vi "receiver.vi"() -> ()   [LabVIEW 2013]
uses:
  <instrlib>/niUSRP/niUSRP Fetch Rx Data (CDB WDT).vi
  <vilib>/express/express analysis/Spectral/Block/exnSpectralBlock spectral measurements RMS poly.vi
  <vilib>/express/express analysis/Spectral/Block/exnSpectralBlock spectral measurements RMS WFM.vi
  <vilib>/express/express analysis/Spectral/XNode/ExpressSpectralMeasurementsBlockNode.xnode
panel:
  out "Waveform Graph 2":cluster{"f0":dbl, "df":dbl, "magnitude":dbl[]}(graph)
  out "Waveform Graph":waveform(dbl)[](graph)
  in  "stop":bool
  out "error out":errorcluster
  in  "number of samples":i64=1000
  out "coerced gain":dbl format="%#_6f"
  out "coerced carrier frequency":dbl=100000.0 format="%#_6p"
  out "coerced IQ rate":dbl=100000.0 format="%#_6p"
  in  "active antenna":string
  in  "gain":dbl format="%#_6f"
  in  "carrier frequency":dbl=100000.0 format="%#_6p"
  in  "IQ rate":dbl=100000.0 format="%#_6p"
  in  "device names":refnum<k15>
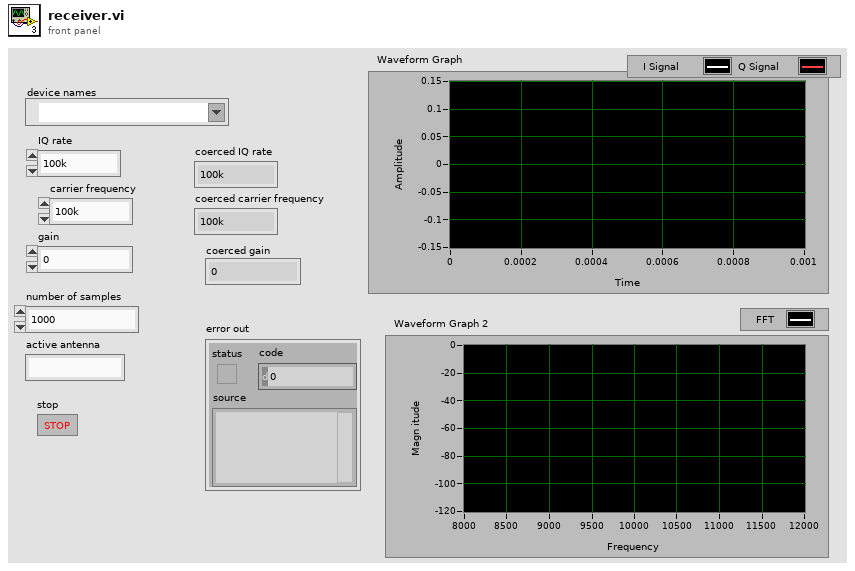
[diagram p1: front panel]
types:
  T1 = cluster{"averaging mode":u16, "weighting mode":u16, "number of averages":u32}
  T2 = cluster{"dB On (F)":bool, "unwrap phase (F)":bool, "convert to degree (F)":bool}
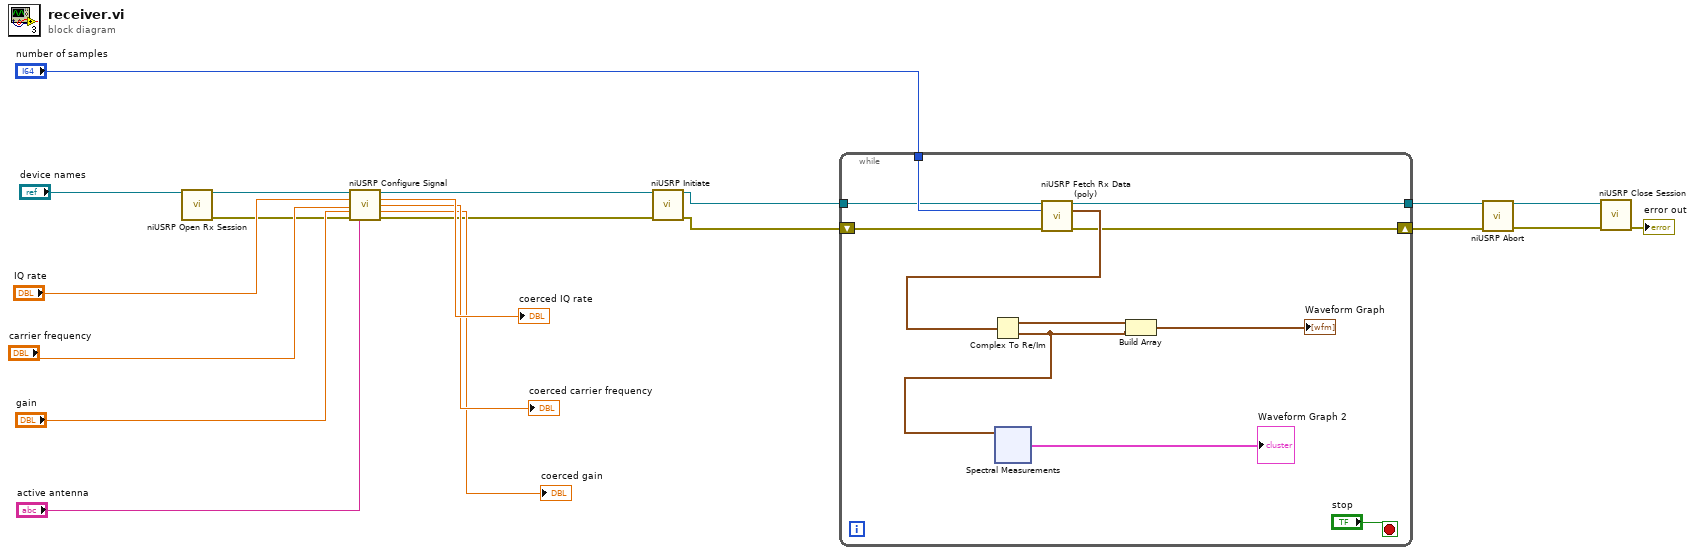
[diagram p0: block diagram]
diagram:
  n1 = call <instrlib>:"niUSRP Open Rx Session.vi"("device names"="device names") -> ("session handle out"=w1:refnum<k15>, "error out"=w2:errorcluster)  [unwired: 13 in]
  n2 = call <instrlib>:"niUSRP Configure Signal.vi"("session handle"=w1, "IQ rate"="IQ rate", "carrier frequency"="carrier frequency", "gain"="gain", "error in (no error)"=w2, "active antenna"="active antenna") -> ("session handle out"=w13:refnum<k15>, "coerced IQ rate"=→"coerced IQ rate":dbl, "coerced carrier frequency"=→"coerced carrier frequency":dbl, "coerced gain"=→"coerced gain":dbl, "error out"=w12:errorcluster)  [unwired: 5 in]
  n3 = call <instrlib>:"niUSRP Initiate.vi"("session handle"=w13, "error in (no error)"=w12) -> ("session handle out"=w10:refnum<k15>, "error out"=w9:errorcluster)  [unwired: 12 in]
  n4 = while {
    tunnel: "number of samples" -> [w31]
    tunnel: w10 -> [w30]
    shift-right: [w26] -> w7
    shift-left: w9 -> [w29]
    tunnel: [w27] -> w8
    stop <- "stop" stop-if-true
    n5 = call-poly <instrlib>:"niUSRP Fetch Rx Data (poly).vi"("session handle"=w30, "number of samples"=w31, "error in (no error)"=w29) -> ("session handle out"=w27:refnum<k15>, "data"=w28:waveform(cdb), "error out"=w26:errorcluster)  [unwired: 9 in, 1 out]
    n6 = Complex To Re/Im(x + iy=w28) -> (x=w24:waveform(dbl), y=w25:waveform(dbl))
    n7 = xnode "Spectral Measurements"("Signals"=w25) -> ("FFT - (RMS)"=→"Waveform Graph 2":cluster{"f0":dbl, "df":dbl, "magnitude":dbl[]})  [unwired: 1 in, 2 out]
    n8 = Build Array(w24, w25) -> (→"Waveform Graph":waveform(dbl)[])
  }
  n9 = call <instrlib>:"niUSRP Abort.vi"("session handle"=w8, "error in (no error)"=w7) -> ("session handle out"=w5:refnum<k15>, "error out"=w6:errorcluster)  [unwired: 12 in]
  n10 = call <instrlib>:"niUSRP Close Session.vi"("session handle"=w5, "error in (no error)"=w6) -> ("error out"=→"error out":errorcluster)  [unwired: 13 in]
